vi "About Dialog.vi"() -> ()   [LabVIEW 2017]
doc: "Show the About Debug Server dialog"
panel:
  out "error out":errorcluster
  in  "error in (no error)":errorcluster
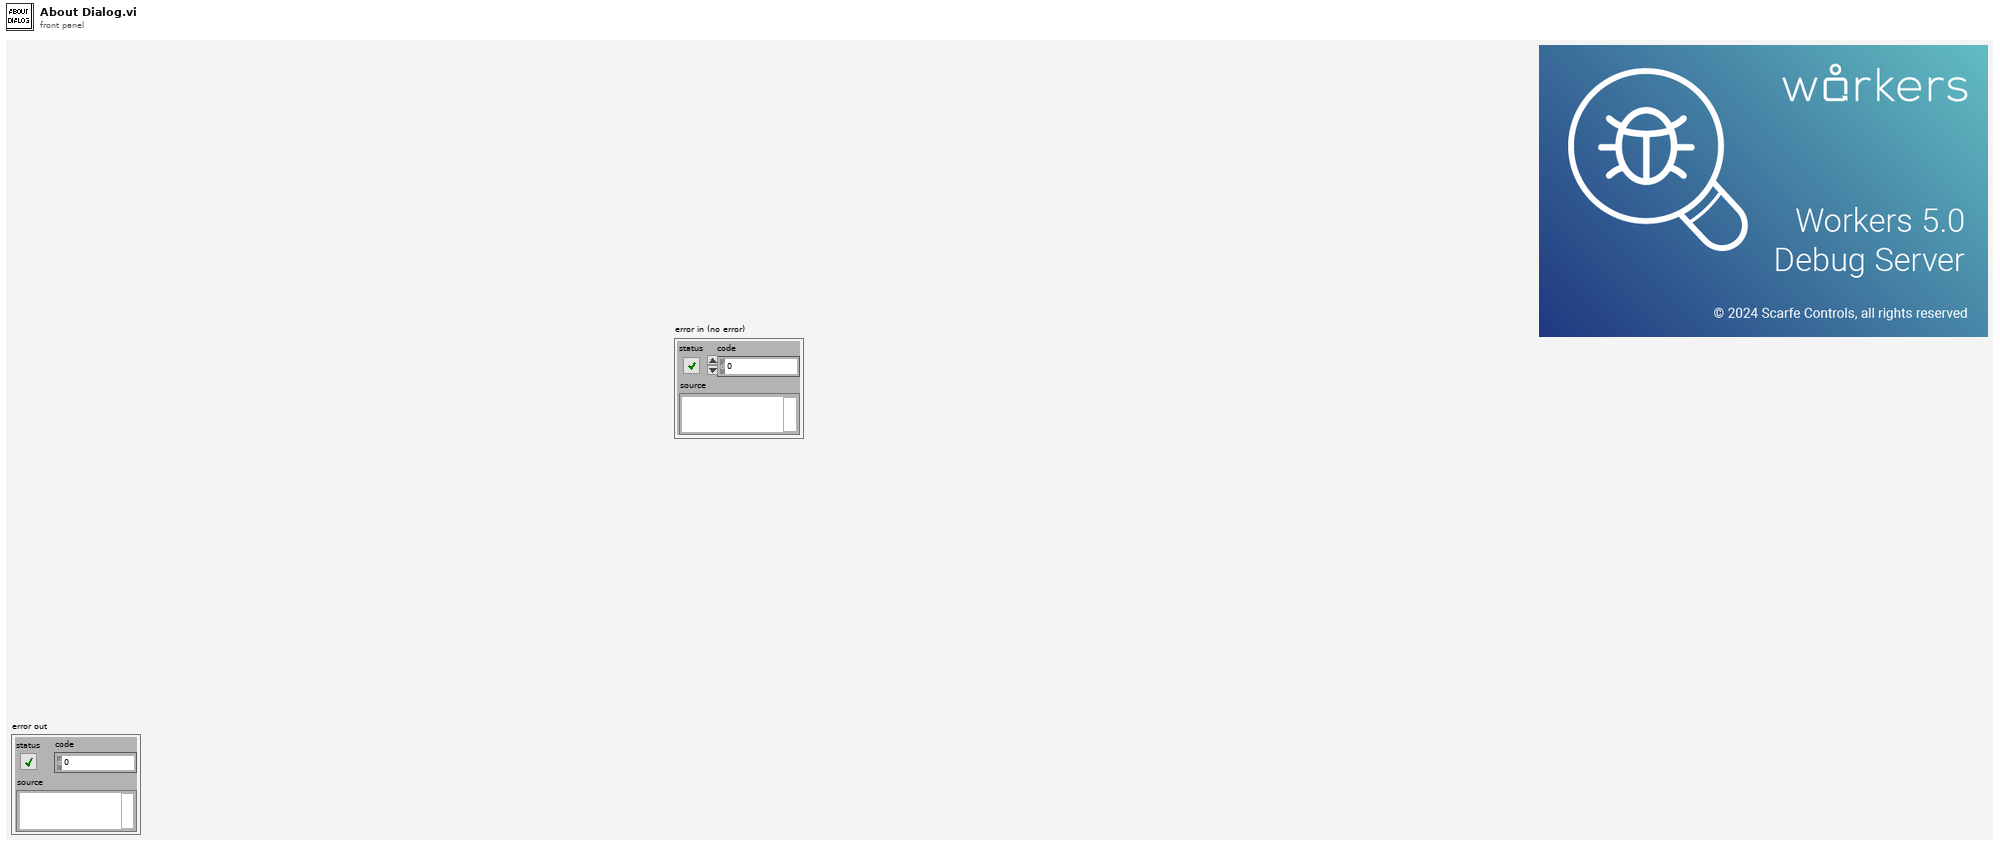
[diagram p1: front panel]
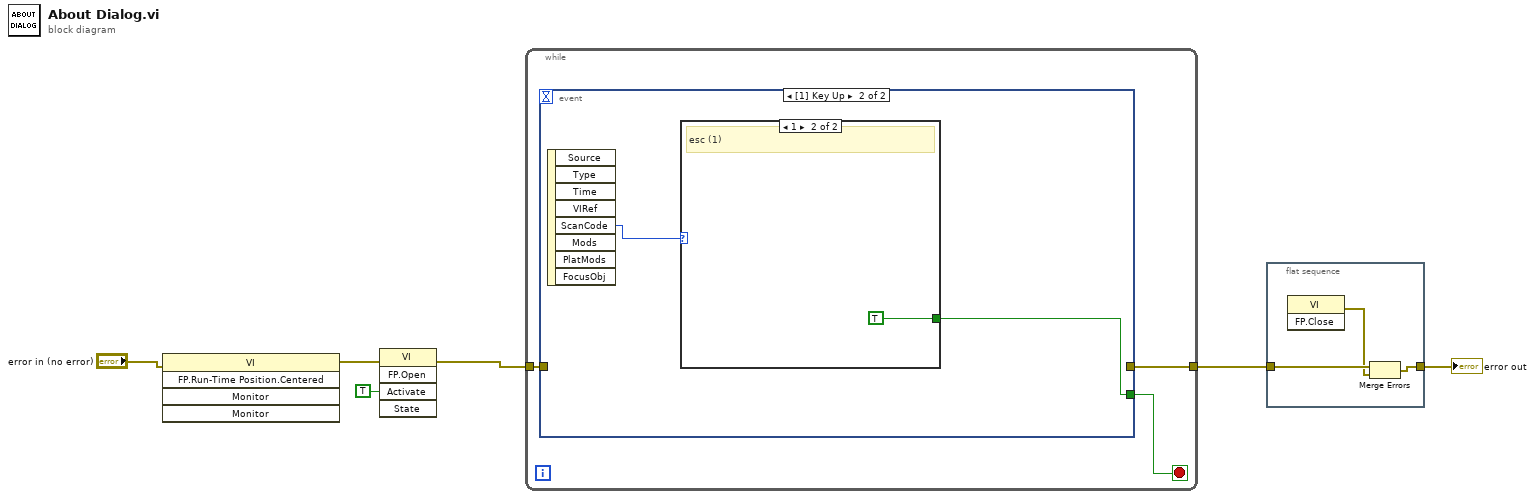
[diagram p0: block diagram]
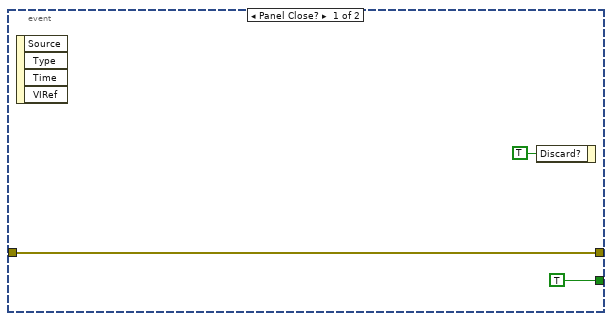
[diagram p2: hidden frame]
diagram:
  n1 = invoke class="VI" method="FP.Run-Time Position.Centered"(error in="error in (no error)") -> (error out=w5:errorcluster)  [unwired: 4 in, 4 out]
  n2 = invoke class="VI" method="FP.Open"(error in=w5, "Activate"=TRUE ("Activate?")) -> (error out=w2:errorcluster)  [unwired: 3 in, 4 out]
  n3 = while {
    tunnel: w2 -> [w8]
    tunnel: [w7] -> w1
    stop <- w9 stop-if-true
    n4 = event shown="[1] Key Up" {
      selector: _ -> [_ _]
      dyn-events: _ -> [_ _]
      timeout: _ -> [_ _]
      tunnel: [TRUE w14] -> w9
      tunnel: w8 -> [w10 _]
      tunnel: [w10 _] -> w7
      event Panel Close? {
        n5 = event-data() -> ()  [unwired: 1 in, 4 out]
        n6 = event-data("Discard?"=TRUE) -> ()  [unwired: 1 in, 1 out]
      }
      event Key Up {
        n7 = event-data() -> ("ScanCode"=w13:i16)  [unwired: 1 in, 7 out]
        n8 = case shown="1" w13 {
          tunnel: [_ TRUE] -> w14
          frame Default {
          }
          frame 1 {
            # "esc (1)"
          }
        }
      }
    }
  }
  n9 = flat-sequence {
    tunnel: [w17] -> w3
    tunnel: w1 -> [w18]
    frame #0 {
      n10 = invoke class="VI" method="FP.Close"() -> (error out=w16:errorcluster)  [unwired: 3 in, 2 out]
      n11 = Merge Errors(w18, w16) -> (w17:errorcluster)
    }
  }
  "error out" <- w3
